vi "StaticBrake Setter.vi"(0 "DeviceReference":T1, 3 "Update Frequency (Hz)":dbl=100.0, 5 "StopSendingOtherRequests":bool=TRUE) -> (4 "DeviceReference Out":T1)   [LabVIEW 2023]
doc: "Applies full neutral-brake by shorting motor leads together."
uses:
  Users/Cory/Documents/PhoenixPro-LabVIEW-Generation/controls/DeviceReference.ctl
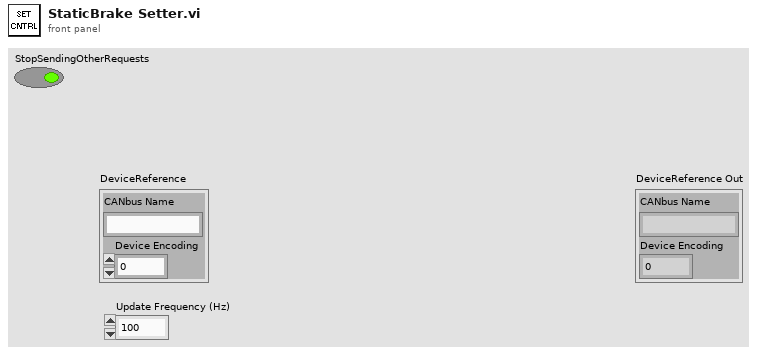
[diagram p1: front panel]
types:
  T1 = typedef "DeviceReference.ctl" = cluster{"CANbus Name":string, "Device Encoding":u32}
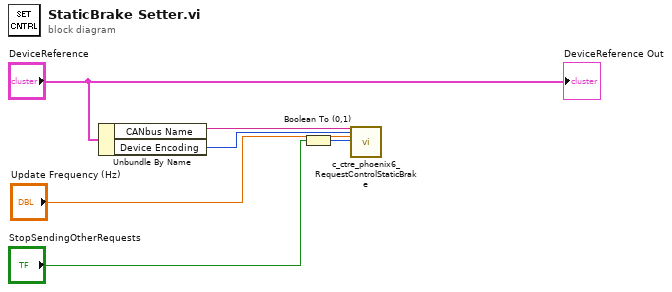
[diagram p0: block diagram]
diagram:
  n1 = Unbundle By Name("DeviceReference") -> ("CANbus Name"=w5:string, "Device Encoding"=w4:u32)
  n2 = Boolean To (0,1)(Boolean="StopSendingOtherRequests") -> (0, 1=w1:i16)
  n3 = call <vilib>:"c_ctre_phoenix6_RequestControlStaticBrake.vi"("String"=w5, "Numeric 2"=w4, "Numeric 3"="Update Frequency (Hz)", "Numeric 4"=w1) -> ()  [unwired: 23 in, 1 out]
  "DeviceReference Out" <- "DeviceReference"
